vi "Close.vi"(8 "error in":errorcluster, 11 "Flow Actual Value in":refnum<class "Flow Actual Value.lvclass">) -> (0 "error out":errorcluster, 3 "Flow Actual Value out":refnum<class "Flow Actual Value.lvclass">)   [LabVIEW 2023, in "Flow Actual Value.lvclass"]
uses:
  Flow Actual Value.lvclass
  Flow Actual Value.lvclass/Flow Actual Value.ctl
  Parents/Actual Value/Actual Value.lvclass
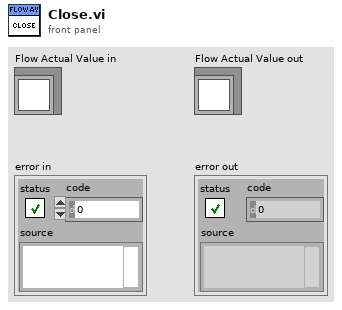
[diagram p1: front panel]
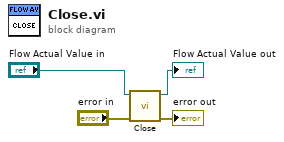
[diagram p0: block diagram]
diagram:
  n1 = call-parent "Close.vi"("error in"="error in", "Actual Value in"="Flow Actual Value in") -> ("error out"=→"error out":errorcluster, "Actual Value out"=→"Flow Actual Value out":refnum<class "Flow Actual Value.lvclass">)  [unwired: 8 in]
